vi "8.0.0_Tester_Functionality_Buyoff.vi"(8 "error in (no error)":errorcluster, 10 "?":T1, 11 "Message Queue out":T2) -> (0 "error out":errorcluster, 1 "Flow":string, 2 "Data":T1, 3 "Message Queue Out":T2)   [LabVIEW 2017]
uses:
  DIPC 692 Daemon API/typdef/calibration.ctl
  DIPC 692 Daemon API/typdef/task_detect_test_point.ctl
  DIPC 692 Daemon API/typdef/device_mode.ctl
  DIPC 692 Daemon API/typdef/destination.ctl
  Depends/AMC/subVIs/TypeDefs/amc_Message Queue.ctl
  Depends/AMC/subVIs/TypeDefs/amc_Message.ctl
  Depends/Tools/Keyed Array/Tools_KeyedArray KeyedArray.ctl
  Ctrls/Data.ctl
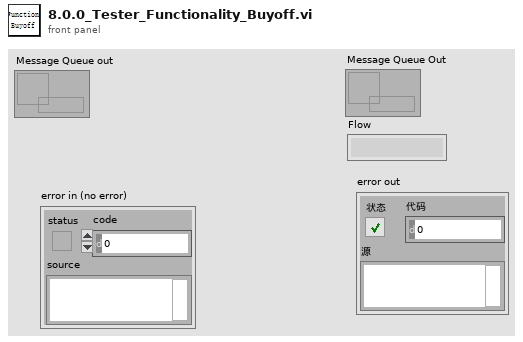
[diagram p1: front panel]
types:
  T1 = typedef "Data.ctl" = cluster{"SN":string, "Start Time":timestamp, "Step Time":timestamp, "Count":cluster{"Total":i32, "OK":i32, "NG":i32, "Yield":dbl}, "Table":string[][], "daemon reference":refnum<k5>, "CT":dbl, "Config":string[][], "Initialisation":cluster{"Set_SKU_Config_With_LMT_Error":string, "FCT_timestamp":string, "sw_version_before":string, "hardware_serial":string, "Backup_DDM_NVM":string, "Flash_SW_follow_SKU":string, "sw_version_after":string, "Set_SKU_Config_base_on_variant":string, "UUT_Ready_Status":string, "Set_DDM_to_EOL_Mode":string, "DDM_Parameter":dbl[], "DDM_Parameter_status":bool[], "Get_Tester_Parameter":dbl[], "Get_Tester_Parameter_status":bool[], "Cal_Tester_Parameter":dbl[], "Cal_Tester_Parameter_status":bool[], "sw_version_before_status":bool, "sw_version_after_status":bool, "Reflashing_Flash_SW_follow_SKU":string, "Set_SKU_Config_With_LMT_status":bool, "FCT_timestamp_status":bool, "LMT_Connect_to_UUT":string, "LMT_Read_SC_SW":string, "LMT_Write_SKU_File":string, "LMT_Connect_to_UUT_status":bool}, "BEMF_Calibration":cluster{"Read_ambient_temperature":dbl, "Set_ambient_temperature_to_DDM":string, "Save_Calibration":string, "Calibration_Vaule":dbl[], "Calibration_Start_Calibration":string, "Calibration_Vaule _B":dbl[], "Calibration_Vaule_status":bool[], "Calibration_Vaule_B_status":bool[], "Orifice_Size":string}, "ECO":cluster{"Reset_Power_tune_vaule_to_zero":string, "ECO_Motor_On_with_power_mode":string, "DDM_Parameter":dbl[], "DDM_Parameter_status":bool[], "Get_Tester_Parameter":dbl[], "Get_Tester_Parameter_status":bool[], "Cal_Tester_Parameter":dbl[], "Cal_Tester_Parameter_status":bool[], "DDM_Parameter_after_power_tune":dbl[], "Get_Tester_Parameter_after_power_tune":dbl[], "Cal_Tester_Parameter_after_power_tune":dbl[], "Cal_Tester_Parameter_after_power_tune_status":bool[], "Delta_P":dbl, "ECO_Power_Tune_Set_Delta_Power_tune_value_to_DDM":string, "ECO_Power_Tune_Motor_On_with_power_mode":string, "Reset_BEMF_FISF_calibration":string, "Orifice_Size":string}, "BOOST":cluster{"DDM_Parameter":dbl[], "DDM_Parameter_status":bool[], "Get_Tester_Parameter":dbl[], "Get_Tester_Parameter_status":bool[], "Cal_Tester_Parameter":dbl[], "Cal_Tester_Parameter_status":bool[], "DDM_Parameter_after_power_tune":dbl[], "Get_Tester_Parameter_after_power_tune":dbl[], "Cal_Tester_Parameter_after_power_tune":dbl[], "Cal_Tester_Parameter_after_power_tune_status":bool[], "airwatts_am_off":dbl, "AW_Delta_(AM_on_and_off)":dbl, "AW_Delta_(AM_on_and_off)_Status":bool, "Delta_P":dbl, "BOOST_Motor_On_with_power_mode":string, "BOOST_Air_Muscle_Check_Turn_off_air_muscle":string, "BOOST_Power_Tune_Set_Delta_Power_tune_value_to_DDM":string, "BOOST_Power_Tune_Motor_On_with_power_mode":string, "BOOST_Stop_motor":string, "BOOST_Save_Calibration":string, "BOOST_Get_AW_Calibration_value":string, "Orifice_Size":string}, "MAX":cluster{"Max_Motor_On_with_power_mode":string, "Average_Tmag_Data":cluster{"LSI Delta in degC":dbl, "FISF Delta in degc":dbl, "LSI Tmag in degC":dbl, "Fisf Tmag in degC":dbl, "IIR Tmag in degC":dbl}, "DDM_Parameter":dbl[], "DDM_Parameter_status":bool[], "Get_Tester_Parameter":dbl[], "Get_Tester_Parameter_status":bool[], "Cal_Tester_Parameter":dbl[], "BEMF_Finetune":cluster{"eol_bemf_mp_cold_coef_c":dbl, "eol_cold_bemf_fisf_offset":dbl}, "AW_Tune":cluster{"delta_P1":dbl, "delta_P_Setting":dbl}, "DDM_Parameter_after_Airwatts_Tune":dbl[], "Get_Tester_Parameter_after_Airwatts_Tune":dbl[], "Cal_Tester_Parameter_after_Airwatts_Tune":dbl[], "DDM_Parameter_after_Airwatts_Finetune":dbl[], "Get_Tester_Parameter_after_Airwatts_Finetune":dbl[], "Cal_Tester_Parameter_after_Airwatts_Finetune":dbl[], "AW_Finetune":cluster{"delta_P2":dbl, "delta_P_Setting":dbl}, "Delta_Tmag_after_tune":cluster{"LSI Delta in degC":dbl, "FISF Delta in degc":dbl, "LSI Tmag in degC":dbl, "Fisf Tmag in degC":dbl, "IIR Tmag in degC":dbl}, "Hot Bemf in mV":dbl, "DDM_Pressure":dbl, "Delta_Pressure":dbl, " Cold Bemf in mV":dbl, " delta Bemf":dbl, " delta p":dbl, "Delta_Pressure_status":bool, " delta Bemf_status":bool, "LSI Delta in degC_status":bool, "FISF Delta in degc_status":bool, "Motor_On_with_power_mode_after_Airwatts_Tune":string, "Airwatts_Finetune_Motor_On_with_power_mode":string, "Airwatts_Finetune_Stop_motor":string, "Max_check_derate_status":string, "Max_Stop_motor":string, "Max_Save_Calibration":string, "Max_check_derate_status_status":bool, "Average_All_data":dbl[][], "Average_Tmag_Data_status":bool[], "Average_Tmag_Data_after_tune_status":bool[], "Orifice_Size":string, "Cal_Tester_Parameter_status":bool[], "Cal_Tester_Parameter_status_after_Airwatts_Tune":bool[], "Cal_Tester_Parameter_status_after_Airwatts_FineTune":bool[]}, "Task_Detect_Calib":cluster{"LL":cluster{"DDM_Parameter":dbl[], "DDM_Parameter_status":bool[], "Get_Tester_Parameter":dbl[], "Get_Tester_Parameter_status":bool[], "Set_task_detect_A":dbl, "LL_Motor_On":string, "Orifice_Size":string, "Set_task_detect_A_Status":bool}, "HL":cluster{"DDM_Parameter":dbl[], "DDM_Parameter_status":bool[], "Get_Tester_Parameter":dbl[], "Get_Tester_Parameter_status":bool[], "Set_task_detect_B":dbl, "HL_Motor_On":string, "HL_Motor_Stop":string, "Set_task_detect_B_Status":bool}, "LH":cluster{"DDM_Parameter":dbl[], "DDM_Parameter_status":bool[], "Get_Tester_Parameter":dbl[], "Get_Tester_Parameter_status":bool[], "Set_task_detect_C":dbl, "LH_Motor_On":string, "Orifice_Size":string, "Set_task_detect_C_Status":bool}, "HH":cluster{"DDM_Parameter":dbl[], "DDM_Parameter_status":bool[], "Get_Tester_Parameter":dbl[], "Get_Tester_Parameter_status":bool[], "Set_task_detect_D":dbl, "HH_Motor_On":string, "HH_Set_calibration_eol_inlet_blockage":string, "HH_Motor_Stop":string, "HH_Save_calibration":string, "Read_and_check_calibration_Status":bool[], "Set_task_detect_D_Status":bool}, "Get_eol_inlet_blockage_E":dbl, "Calib_vaule":cluster{"Get_task_detect_LL":dbl, "Get_task_detect_HL":dbl, "Get_task_detect_LH":dbl, "Get_task_detect_HH":dbl, "eol_inlet_blockage":dbl, "eol_code_bemf_temp":dbl}, "Reset_all_task_detect_calibration_parameter":string, "calibrated temp":dbl, "Set ambient temperature to DDM":string, "Set ambient temperature to DDM after task detect":string, "Inlet_Blockage_Calibration":cluster{"DDM_Parameter":dbl[], "DDM_Parameter_status":bool[], "Get_Tester_Parameter":dbl[], "Get_Tester_Parameter_status":bool[], "Inlet_Blockage_Calibration_Motor_On":string, "Calibrate Inlet Blockage":string}, "Get_eol_inlet_blockage_E_Status":bool}, "good":cluster{"Write_Product_TS":cluster{"TIMESTAMP":i64, "RIG_ID":i64, "PASSMARK_ID":i64, "PASSMARK_REV":i64}, "Read_Product_TS":cluster{"TIMESTAMP":i64, "RIG_ID":i64, "PASSMARK_ID":i64, "PASSMARK_REV":i64}, "Good_Clear_NVM_Error":string, "Good_Set_DDM_to_Product_mode":string, "Good_Write_Product_Timestamp":string, "Good_Read_Product_Timestamp":string, "Good_Backup_DDM_NVM":string, "Good_Set_Secuity_Bit":string, "Good_Set_Calibration_Lock":string, "Good_Check_Secuity_Bit":string, "Good_Check_Secuity_Bit_Stauts":bool}, "UUT_Type":enum16{"692", "692B", "692D"}, "NG":cluster{"NG_Read_Error":string, "NG_Change_to_FCT_mode":string, "NG_Backup_DDM_NVM":string}, "OK/NG":bool, "Model":string, "Station ID":string}
  T2 = typedef "amc_Message Queue.ctl" = refnum<queue>
  T3 = typedef "HD Config.ctl" = cluster{" PC":cluster{"PC Address":u8[], "PC Port":i32}, "FCO":cluster{"COM":refnum<visa-resource-name>, "Baudrate":u32}, "DC Power ":cluster{"COM":refnum<visa-resource-name>, "Baudrate":u32}, "PW3336":cluster{"COM":refnum<visa-resource-name>, "Baudrate":u32}, "Lefoo":cluster{"COM":refnum<visa-resource-name>, "Baudrate":u32}, "AI Model":cluster{"COM":refnum<visa-resource-name>, "Baudrate":u32}, "DIPC":cluster{"COM":refnum<visa-resource-name>}, "Daemon":cluster{"IP Address":string, "Port":u16, "Retry":u16}, "Motor":cluster{"COM":refnum<visa-resource-name>, "Baudrate":u32}, "G1":bool, "Fail_resume_mode":bool, "Skip DDM Speed&Pressure Passmark":bool}
  T4 = typedef "destination.ctl" = string
  T5 = typedef "calibration.ctl" = string
  T6 = typedef "device_mode.ctl" = enum16{"FCT", "EOL", "PROD"}
  T7 = typedef "airwatt tune parameter.ctl" = cluster{"Index(0-5)":i64, "Target power mW":i64, "Offset power mW":i64}
  T8 = typedef "task_detect_test_point.ctl" = enum16{"LL", "HL", "LH", "HH"}
  T9 = cluster{"TIMESTAMP":i64, "RIG_ID":i64, "PASSMARK_ID":i64, "PASSMARK_REV":i64}
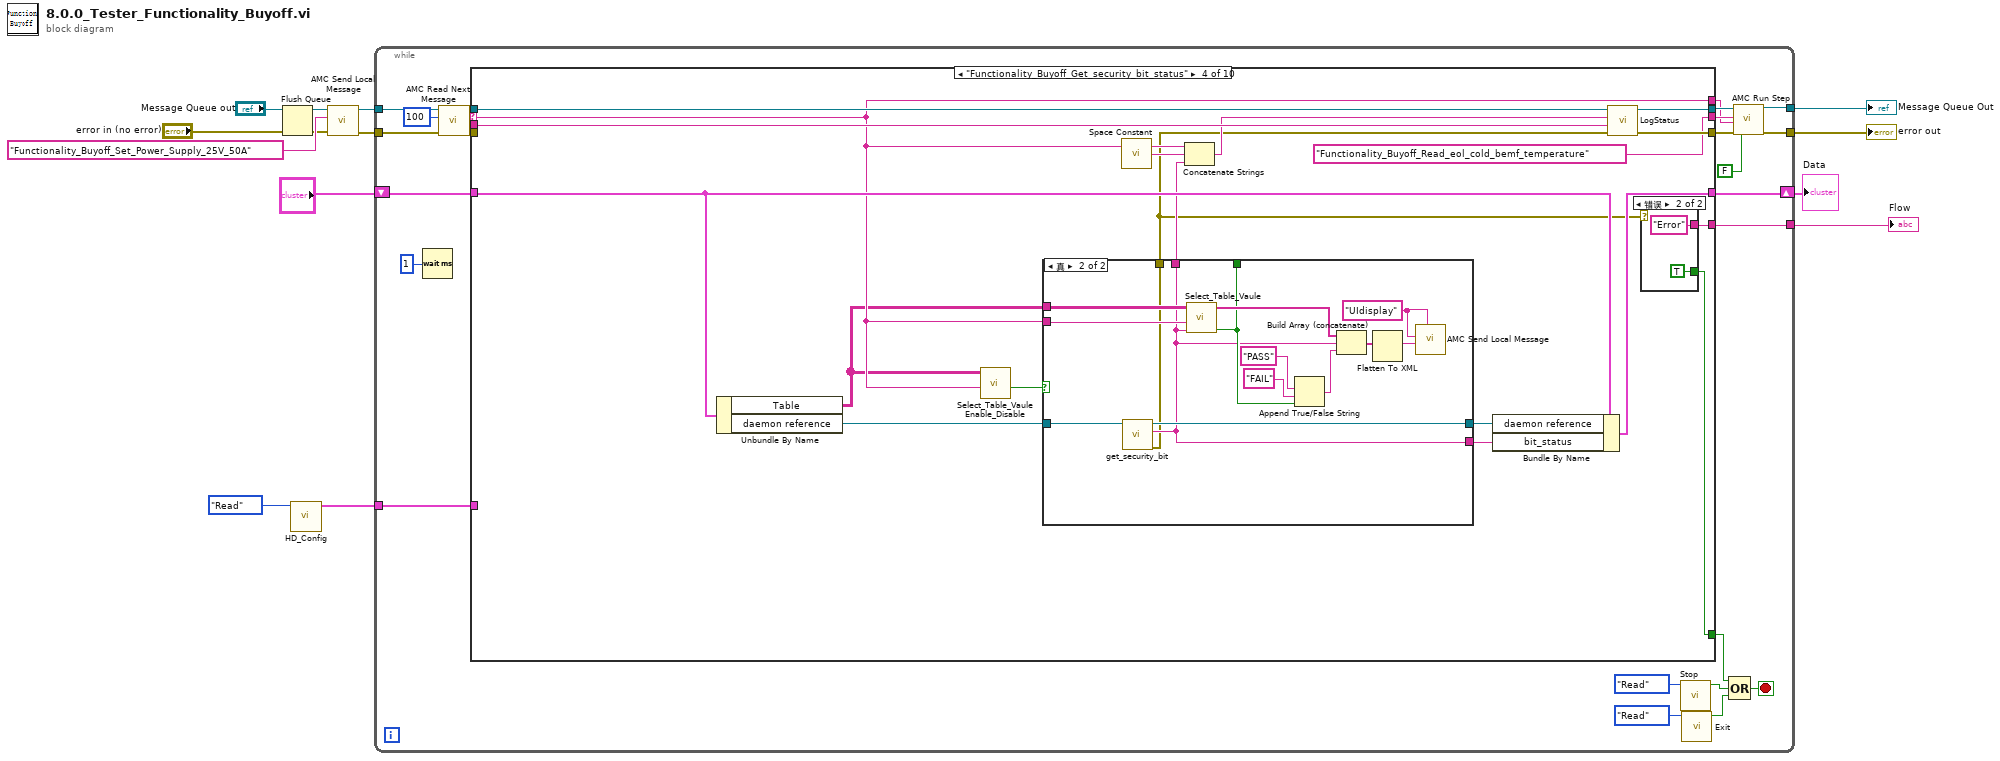
[diagram p0: block diagram]
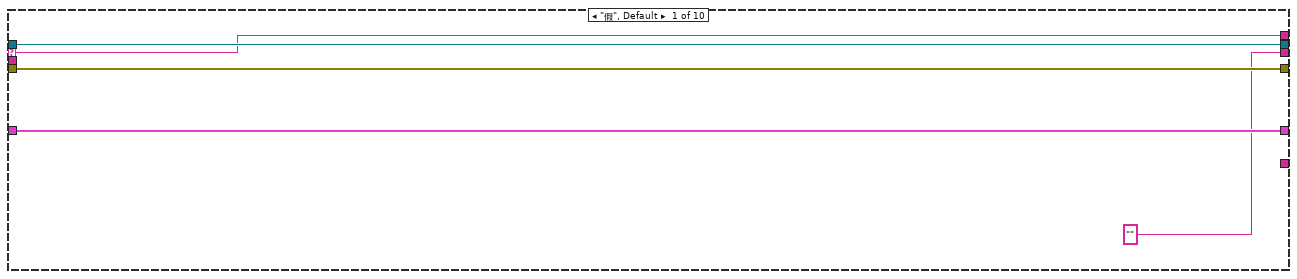
[diagram p2: hidden frame]
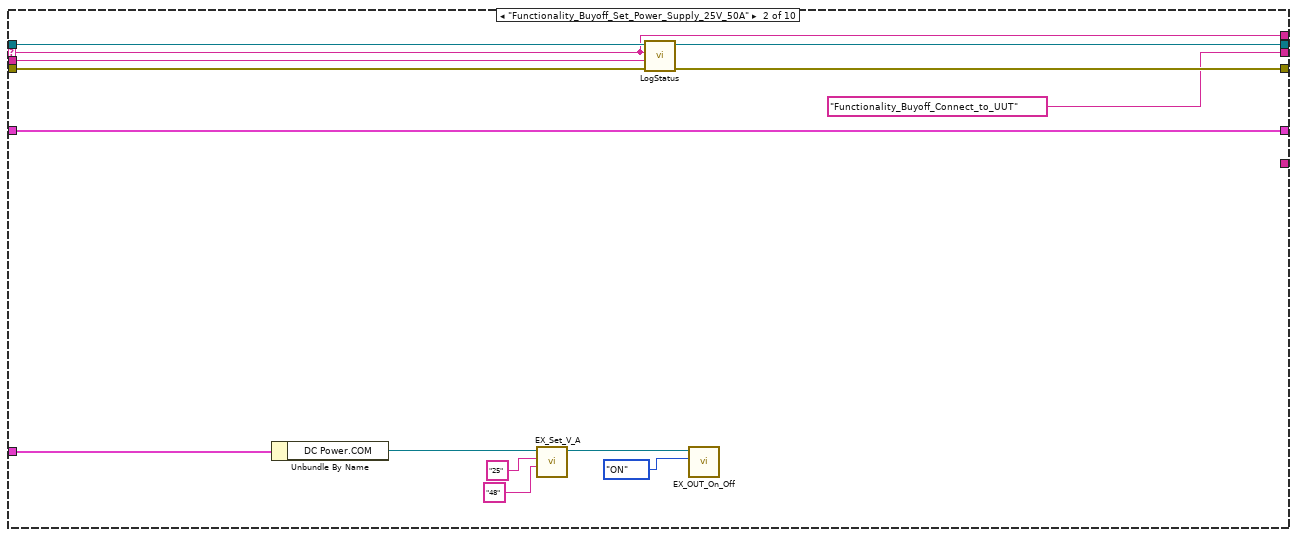
[diagram p3: hidden frame]
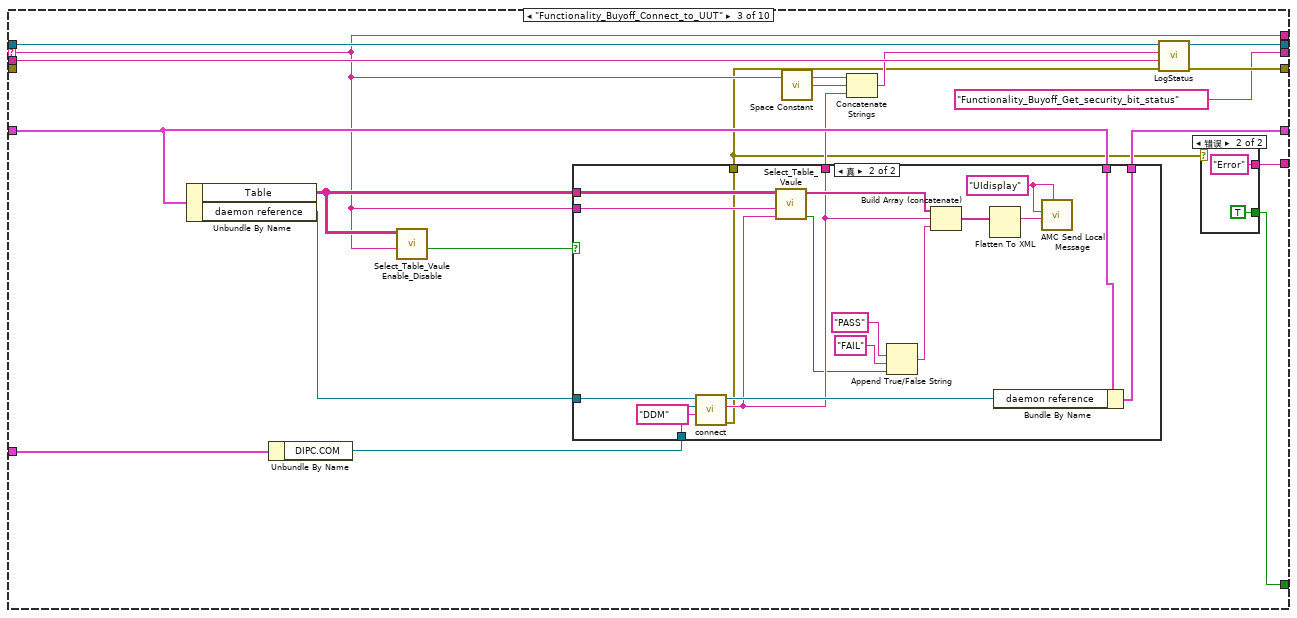
[diagram p4: hidden frame]
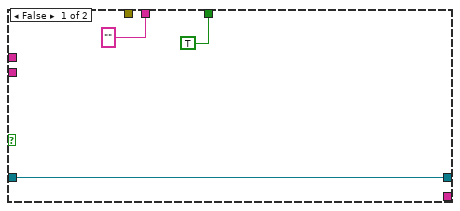
[diagram p8: hidden frame]
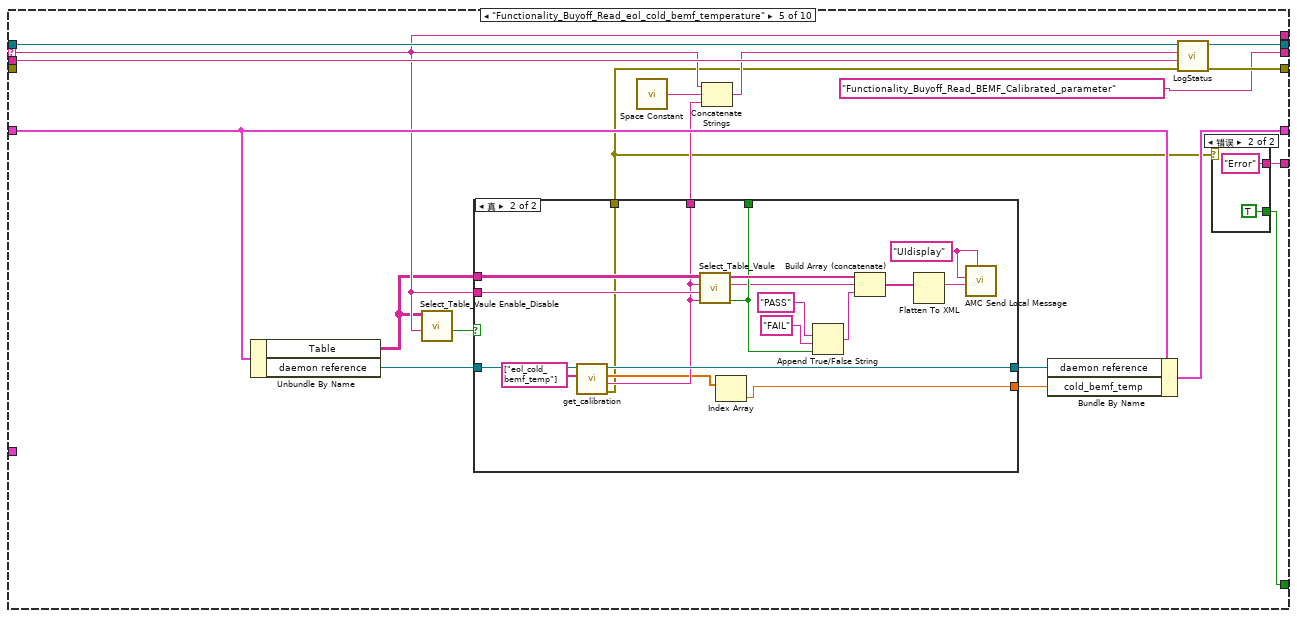
[diagram p9: hidden frame]
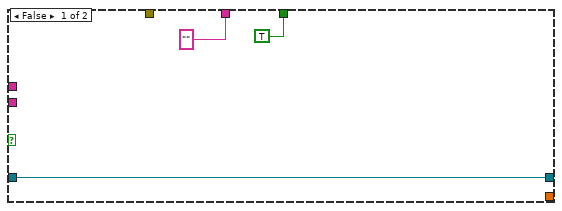
[diagram p11: hidden frame]
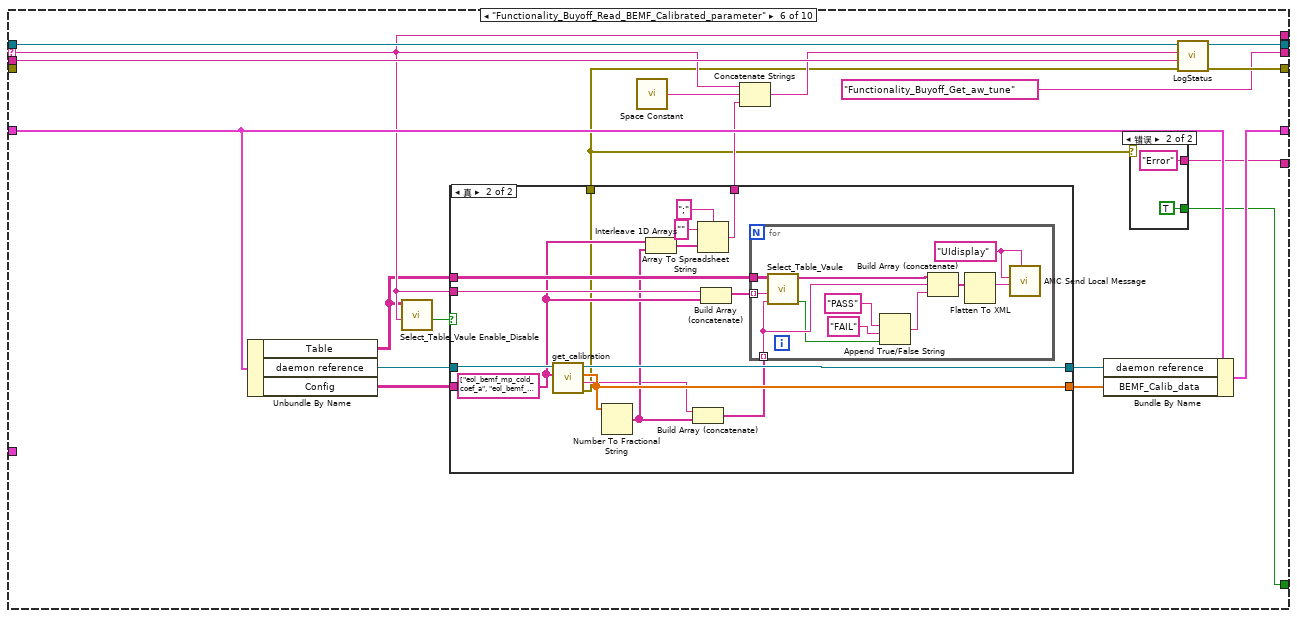
[diagram p12: hidden frame]
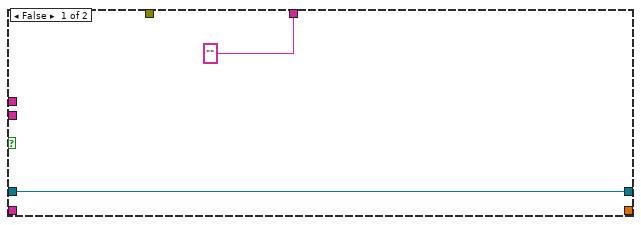
[diagram p14: hidden frame]
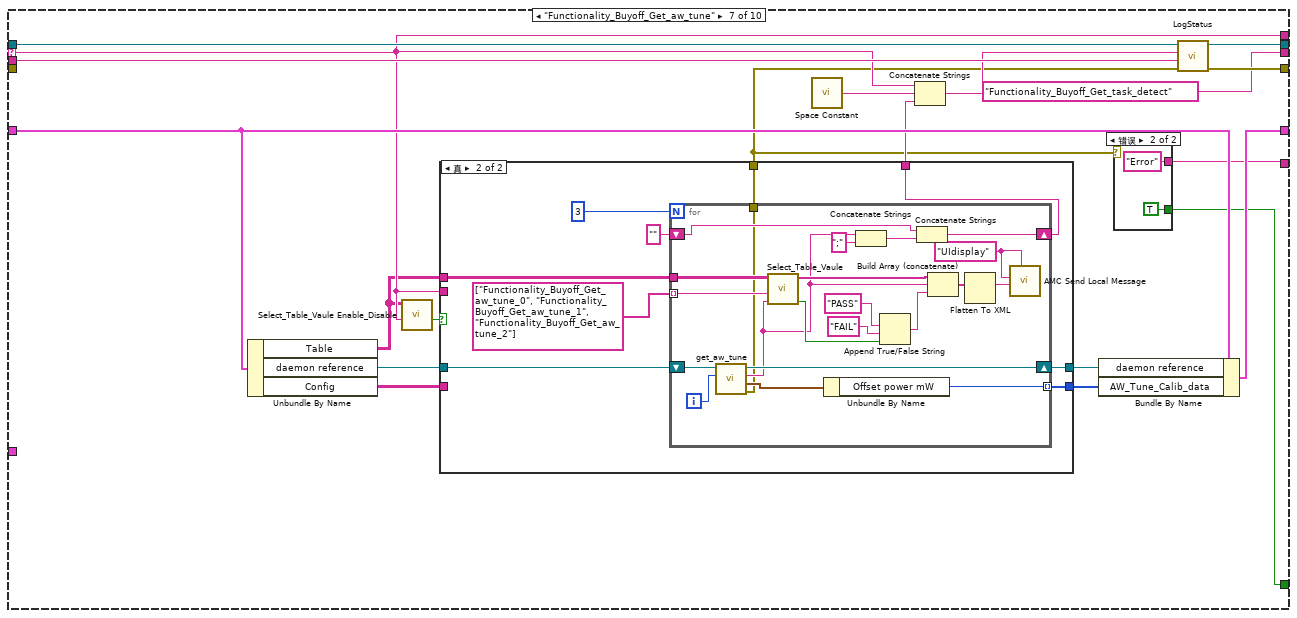
[diagram p15: hidden frame]
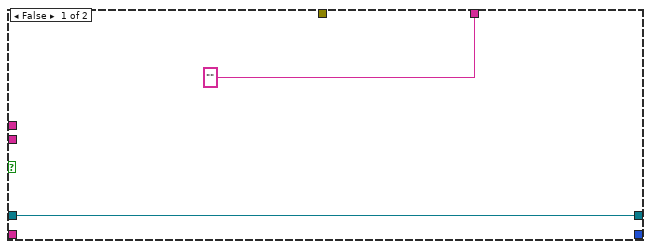
[diagram p17: hidden frame]
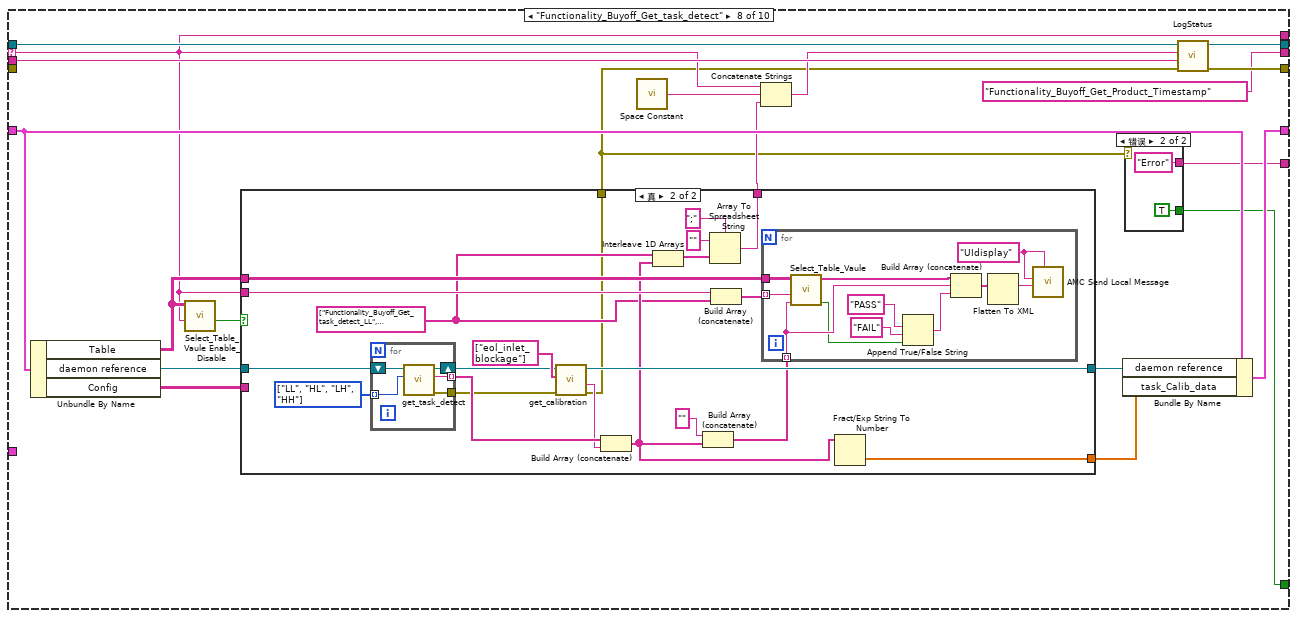
[diagram p18: hidden frame]
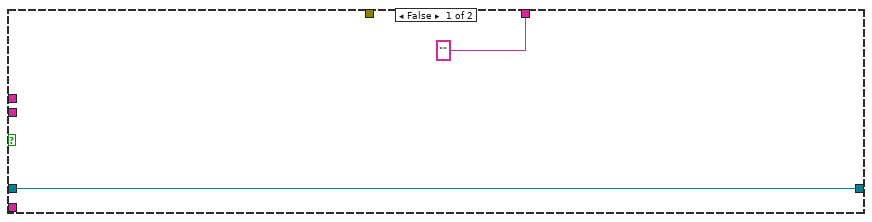
[diagram p20: hidden frame]
diagram:
  n1 = Flush Queue(queue="Message Queue out") -> (queue out=w1:T2)  [unwired: 1 in, 2 out]
  n2 = call "HD_Config.vi"("Step"=enum16{"Initial", "Write", "Read"}."Read") -> ("HD Config out"=w5:T3)  [unwired: 9 in, 1 out]
  n3 = call "AMC Send Local Message.vi"("error in (no error)"="error in (no error)", "Message Name"="Functionality_Buyoff_Set_Power_Supply_25V_50A", "Message Queue in"=w1) -> ("error out"=w10:errorcluster, "Message Queue out"=w11:T2)  [unwired: 7 in]
  n4 = while {
    tunnel: w11 -> [w38]
    tunnel: [w34] -> w3
    tunnel: w10 -> [w32]
    tunnel: [w29] -> w2
    shift-right: [w25] -> w7
    shift-left: "?" -> [w26]
    tunnel: w5 -> [w24]
    tunnel: [w20] -> w4
    stop <- w14 stop-if-true
    n5 = Wait (ms)(milliseconds to wait=u32 1 ("等待时间（毫秒）")) -> ()  [unwired: 1 out]
    n6 = call "AMC Read Next Message.vi"("error in (no error)"=w32, "timeout (1ms)"=100, "Message Queue in"=w38) -> ("error out"=w31:errorcluster, "Message Value"=w22:string, "Message Name"=w36:string, "Message Queue out"=w37:T2)  [unwired: 1 in, 4 out]
    n7 = case shown="\"Functionality_Buyoff_Get_security_bit_status\"" w36 {
      selector: w36 -> [w40 w51 w62 w102 w139 w181 w230 w281 w342 w379]
      tunnel: w37 -> [w43 w56 w74 w113 w150 w191 w240 w293 w352 w390]
      tunnel: [w43 w56 w74 w113 w150 w191 w240 w293 w352 w390] -> w35
      tunnel: w31 -> [w42 w54 _ _ _ _ _ _ _ _]
      tunnel: [w42 w53 w73 w112 w149 w190 w239 w292 w351 w389] -> w30
      tunnel: [_ _ w59 w97 w134 w174 w223 w276 w336 TRUE] -> w15
      tunnel: w26 -> [w41 w55 w67 w108 w146 w187 w236 w290 w348 w386]
      tunnel: [w41 w55 w68 w107 w145 w186 w235 w289 w347 w385] -> w25
      tunnel: w22 -> [_ w52 w72 w111 w148 w189 w238 w291 w350 w388]
      tunnel: [w40 w51 w62 w102 w139 w181 w230 w281 w342 w379] -> w21
      tunnel: w24 -> [_ w45 w70 _ _ _ _ _ _ _]
      tunnel: ["" "Functionality_Buyoff_Connect_to_UUT" "Functionality_Buyoff_Get_security_bit_status" "Functionality_Buyoff_Read_eol_cold_bemf_temperature" "Functionality_Buyoff_Read_BEMF_Calibrated_parameter" "Functionality_Buyoff_Get_aw_tune" "Functionality_Buyoff_Get_task_detect" "Functionality_Buyoff_Get_Product_Timestamp" "Functionality_Buyoff_Get_calibration_lock_status" w376] -> w23
      tunnel: [_ _ w60 w98 w135 w175 w224 w277 w338 w376] -> w20
      frame "假", Default {
      }
      frame "Functionality_Buyoff_Set_Power_Supply_25V_50A" {
        n8 = Unbundle By Name(w45) -> ("DC Power.COM"=w44:refnum<visa-resource-name>)
        n9 = call "EX_Set_V_A.vi"("current"="48", "voltage"="25", "VISA resource name"=w44) -> ("VISA资源名称输出"=w47:refnum<visa-resource-name>)  [unwired: 7 in, 1 out]
        n10 = call "LogStatus.vi"("error in (no error)"=w54, "last message"=w52, "message"=w51) -> ("error  out"=w53:errorcluster)  [unwired: 8 in]
        n11 = call "EX_OUT_On_Off.vi"("Mode"=enum16{"ON", "OFF"}."ON", "VISA resource name"=w47) -> ()  [unwired: 8 in, 2 out]
      }
      frame "Functionality_Buyoff_Connect_to_UUT" {
        n12 = Unbundle By Name(w67) -> ("Table"=w63:string[][], "daemon reference"=w57:refnum<k5>)
        n13 = Unbundle By Name(w70) -> ("DIPC.COM"=w69:refnum<visa-resource-name>)
        n14 = call "Select_Table_Vaule Enable_Disable.vi"("Action"=w62, "Table"=w63) -> ("Enable"=w61:bool)  [unwired: 8 in, 1 out]
        n15 = case shown="真" w61 {
          tunnel: w69 -> [_ w95]
          tunnel: [w77 w94] -> w68
          tunnel: w67 -> [w77 w93]
          tunnel: [_ w84] -> w64
          tunnel: w63 -> [_ w82]
          tunnel: w62 -> [_ w81]
          tunnel: [_ w80] -> w58
          tunnel: w57 -> [_ w79]
          frame False {
          }
          frame True {
            w90 = "UIdisplay" ("Process (\"\" - local)")
            n16 = call "connect.vi"("Target"=T4 "DDM", "physical connection"=w95, "daemon reference in"=w79) -> ("error out"=w80:errorcluster, "response"=w84:string, "daemon reference out"=w91:refnum<k5>)  [unwired: 4 in, 2 out]
            n17 = call "Select_Table_Vaule.vi"("Vaule"=w84, "Action"=w81, "Table"=w82) -> ("Result"=w83:bool, "vaule"=w92:string[])  [unwired: 7 in]
            n18 = Append True/False String(1:w83, 2:"FAIL" ("真字符串"), 3:"PASS" ("真字符串")) -> (0:w85:string)  [unwired: 1 in]
            n19 = Build Array (concatenate)(w92, w84, w85) -> (w89:string[])
            n20 = Flatten To XML(anything=w89) -> (xml string=w88:string)
            n21 = Bundle By Name(cluster=w93, "daemon reference"=w91) -> (w94:T1)
            n22 = call "AMC Send Local Message.vi"("Process (\"\" - local)"=w90, "Message Value"=w88, "Message Name"=w90) -> ()  [unwired: 7 in, 2 out]
          }
        }
        n23 = call <vilib>:"Space Constant.vi"() -> ("String"=w65:string)
        n24 = Concatenate Strings(w62, w65, w64) -> (w66:string)
        n25 = call "LogStatus.vi"("error in (no error)"=w58, "last message"=w72, "message"=w66) -> ("error  out"=w73:errorcluster)  [unwired: 8 in]
        n26 = case shown="错误" w58 {
          tunnel: [_ TRUE] -> w59
          tunnel: [_ "Error"] -> w60
          frame No Error {
          }
          frame Error {
          }
        }
      }
      frame "Functionality_Buyoff_Get_security_bit_status" {
        n27 = Unbundle By Name(w108) -> ("Table"=w101:string[][], "daemon reference"=w110:refnum<k5>)
        n28 = call "Select_Table_Vaule Enable_Disable.vi"("Action"=w102, "Table"=w101) -> ("Enable"=w103:bool)  [unwired: 8 in, 1 out]
        n29 = case shown="真" w103 {
          tunnel: w110 -> [w117 w132]
          tunnel: [TRUE w121] -> _
          tunnel: [w117 w125] -> w109
          tunnel: ["" ("response") w120] -> w104
          tunnel: w102 -> [_ w124]
          tunnel: w101 -> [_ w123]
          tunnel: [_ w120] -> w99
          tunnel: [_ w119] -> w96
          frame False {
          }
          frame True {
            w131 = "UIdisplay" ("Process (\"\" - local)")
            n30 = call "get_security_bit.vi"("daemon reference in"=w132) -> ("error out"=w119:errorcluster, "response"=w120:string, "daemon reference out"=w125:refnum<k5>)  [unwired: 7 in, 1 out]
            n31 = call "Select_Table_Vaule.vi"("Vaule"=w120, "Action"=w124, "Table"=w123) -> ("Result"=w121:bool, "vaule"=w122:string[])  [unwired: 7 in]
            n32 = Append True/False String(1:w121, 2:"FAIL" ("真字符串"), 3:"PASS" ("真字符串")) -> (0:w126:string)  [unwired: 1 in]
            n33 = Build Array (concatenate)(w122, w120, w126) -> (w130:string[])
            n34 = Flatten To XML(anything=w130) -> (xml string=w129:string)
            n35 = call "AMC Send Local Message.vi"("Process (\"\" - local)"=w131, "Message Value"=w129, "Message Name"=w131) -> ()  [unwired: 7 in, 2 out]
          }
        }
        n36 = call <vilib>:"Space Constant.vi"() -> ("String"=w106:string)
        n37 = Concatenate Strings(w102, w106, w104) -> (w105:string)
        n38 = Bundle By Name(cluster=w108, "daemon reference"=w109, "bit_status"=w99) -> (w107:T1)
        n39 = call "LogStatus.vi"("error in (no error)"=w96, "last message"=w111, "message"=w105) -> ("error  out"=w112:errorcluster)  [unwired: 8 in]
        n40 = case shown="错误" w96 {
          tunnel: [_ TRUE] -> w97
          tunnel: [_ "Error"] -> w98
          frame No Error {
          }
          frame Error {
          }
        }
      }
      frame "Functionality_Buyoff_Read_eol_cold_bemf_temperature" {
        n41 = Unbundle By Name(w146) -> ("Table"=w138:string[][], "daemon reference"=w147:refnum<k5>)
        n42 = call "Select_Table_Vaule Enable_Disable.vi"("Action"=w139, "Table"=w138) -> ("Enable"=w140:bool)  [unwired: 8 in, 1 out]
        n43 = case shown="真" w140 {
          tunnel: w147 -> [w154 w166]
          tunnel: [TRUE w161] -> _
          tunnel: [w154 w165] -> w144
          tunnel: ["" ("software string") w159] -> w141
          tunnel: w139 -> [_ w164]
          tunnel: w138 -> [_ w163]
          tunnel: [_ w157] -> w136
          tunnel: [_ w156] -> w133
          frame False {
          }
          frame True {
            w172 = "UIdisplay" ("Process (\"\" - local)")
            n44 = call "get_calibration.vi"("Calibration"=T5[] ["eol_cold_bemf_temp"], "daemon reference in"=w166) -> ("error out"=w156:errorcluster, "response"=w159:string, "values"=w158:dbl[], "daemon reference out"=w165:refnum<k5>)  [unwired: 5 in, 1 out]
            n45 = call "Select_Table_Vaule.vi"("Vaule"=w159, "Action"=w164, "Table"=w163) -> ("Result"=w161:bool, "vaule"=w162:string[])  [unwired: 7 in]
            n46 = Index Array(array=w158) -> (element=w157:dbl)  [unwired: 1 in]
            n47 = Append True/False String(1:w161, 2:"FAIL" ("真字符串"), 3:"PASS" ("真字符串")) -> (0:w167:string)  [unwired: 1 in]
            n48 = Build Array (concatenate)(w162, w159, w167) -> (w171:string[])
            n49 = Flatten To XML(anything=w171) -> (xml string=w170:string)
            n50 = call "AMC Send Local Message.vi"("Process (\"\" - local)"=w172, "Message Value"=w170, "Message Name"=w172) -> ()  [unwired: 7 in, 2 out]
          }
        }
        n51 = call <vilib>:"Space Constant.vi"() -> ("String"=w143:string)
        n52 = Concatenate Strings(w139, w143, w141) -> (w142:string)
        n53 = Bundle By Name(cluster=w146, "daemon reference"=w144, "cold_bemf_temp"=w136) -> (w145:T1)
        n54 = call "LogStatus.vi"("error in (no error)"=w133, "last message"=w148, "message"=w142) -> ("error  out"=w149:errorcluster)  [unwired: 8 in]
        n55 = case shown="错误" w133 {
          tunnel: [_ TRUE] -> w134
          tunnel: [_ "Error"] -> w135
          frame No Error {
          }
          frame Error {
          }
        }
      }
      frame "Functionality_Buyoff_Read_BEMF_Calibrated_parameter" {
        n56 = Unbundle By Name(w187) -> ("Table"=w180:string[][], "daemon reference"=w188:refnum<k5>, "Config"=w178:string[][])
        n57 = call "Select_Table_Vaule Enable_Disable.vi"("Action"=w181, "Table"=w180) -> ("Enable"=w179:bool)  [unwired: 8 in, 1 out]
        n58 = case shown="真" w179 {
          tunnel: w188 -> [w195 w209]
          tunnel: [w195 w208] -> w185
          tunnel: ["" ("software string") w199] -> w182
          tunnel: w181 -> [_ w206]
          tunnel: w180 -> [_ w210]
          tunnel: w178 -> [_ _]
          tunnel: [_ w207] -> w176
          tunnel: [_ w196] -> w173
          frame False {
          }
          frame True {
            w204 = T5[] ["eol_bemf_mp_cold_coef_a", "eol_bemf_mp_cold_coef_b", "eol_bemf_mp_cold_coef_c", "eol_bemf_lsi_cold_ref_coeffs", "eol_bemf_lsi_speed", "eol_bemf_lsi_integral_0", "eol_bemf_lsi_integral_1", "eol_bemf_lsi_integral_2", "eol_cold_bemf", "eol_cold_bemf_fisf", "eol_cold_bemf_fisf_offset"] ("Calibration")
            n59 = call "get_calibration.vi"("Calibration"=w204, "daemon reference in"=w209) -> ("error out"=w196:errorcluster, "response"=w201:string, "values"=w207:dbl[], "daemon reference out"=w208:refnum<k5>)  [unwired: 5 in, 1 out]
            n60 = Number To Fractional String(number=w207) -> (F-format string=w203:string[])  [unwired: 3 in]
            n61 = Interleave 1D Arrays(w204, w203) -> (w200:T5[])
            n62 = Build Array (concatenate)(w201, w203) -> (w202:string[])
            n63 = Array To Spreadsheet String(delimiter (Tab)=";" ("分隔符(Tab)"), array=w200, 3:"" ("格式字符串")) -> (spreadsheet string=w199:string)
            n64 = Build Array (concatenate)(w206, w204) -> (w205:T5[])
            n65 = for {
              tunnel: w210 -> [w215]
              tunnel: w202 -> [w213] mode=indexing
              tunnel: w205 -> [w212] mode=indexing
              w221 = "UIdisplay" ("Process (\"\" - local)")
              n66 = call "Select_Table_Vaule.vi"("Vaule"=w213, "Action"=w212, "Table"=w215) -> ("Result"=w211:bool, "vaule"=w214:string[])  [unwired: 7 in]
              n67 = Append True/False String(1:w211, 2:"FAIL" ("真字符串"), 3:"PASS" ("真字符串")) -> (0:w216:string)  [unwired: 1 in]
              n68 = Build Array (concatenate)(w214, w213, w216) -> (w220:string[])
              n69 = Flatten To XML(anything=w220) -> (xml string=w219:string)
              n70 = call "AMC Send Local Message.vi"("Process (\"\" - local)"=w221, "Message Value"=w219, "Message Name"=w221) -> ()  [unwired: 7 in, 2 out]
            }
          }
        }
        n71 = call <vilib>:"Space Constant.vi"() -> ("String"=w184:string)
        n72 = Concatenate Strings(w181, w184, w182) -> (w183:string)
        n73 = Bundle By Name(cluster=w187, "daemon reference"=w185, "BEMF_Calib_data"=w176) -> (w186:T1)
        n74 = case shown="错误" w173 {
          tunnel: [_ TRUE] -> w174
          tunnel: [_ "Error"] -> w175
          frame No Error {
          }
          frame Error {
          }
        }
        n75 = call "LogStatus.vi"("error in (no error)"=w173, "last message"=w189, "message"=w183) -> ("error  out"=w190:errorcluster)  [unwired: 8 in]
      }
      frame "Functionality_Buyoff_Get_aw_tune" {
        n76 = Unbundle By Name(w236) -> ("Table"=w229:string[][], "daemon reference"=w237:refnum<k5>, "Config"=w227:string[][])
        n77 = call "Select_Table_Vaule Enable_Disable.vi"("Action"=w230, "Table"=w229) -> ("Enable"=w228:bool)  [unwired: 8 in, 1 out]
        n78 = case shown="真" w228 {
          tunnel: w237 -> [w244 w252]
          tunnel: [w244 w251] -> w234
          tunnel: ["" ("software string") w246] -> w231
          tunnel: w230 -> [_ _]
          tunnel: w229 -> [_ w253]
          tunnel: w227 -> [_ _]
          tunnel: [_ w248] -> w225
          tunnel: [_ w245] -> w222
          frame False {
          }
          frame True {
            n79 = for {
              N: 3 -> [_]
              tunnel: w253 -> [w274]
              shift-right: [w272] -> w251
              shift-left: w252 -> [w273]
              tunnel: string[] ["Functionality_Buyoff_Get_aw_tune_0", "Functionality_Buyoff_Get_aw_tune_1", "Functionality_Buyoff_Get_aw_tune_2"] -> [w262] mode=indexing
              tunnel: [w260] -> w248 mode=indexing
              shift-right: [w257] -> w246
              shift-left: "" -> [w256]
              tunnel: [w254] -> w245
              i -> [w263]
              w271 = "UIdisplay" ("Process (\"\" - local)")
              n80 = call "get_aw_tune.vi"("Index"=w263, "daemon reference in"=w273) -> ("error out"=w254:errorcluster, "AW Tune Parameter"=w261:T7, "response"=w259:string, "daemon reference out"=w272:refnum<k5>)  [unwired: 5 in, 1 out]
              n81 = call "Select_Table_Vaule.vi"("Vaule"=w259, "Action"=w262, "Table"=w274) -> ("Result"=w264:bool, "vaule"=w265:string[])  [unwired: 7 in]
              n82 = Unbundle By Name(w261) -> ("Offset power mW"=w260:i64)
              n83 = Concatenate Strings(w259, ";" ("字符串")) -> (w255:string)
              n84 = Append True/False String(1:w264, 2:"FAIL" ("真字符串"), 3:"PASS" ("真字符串")) -> (0:w266:string)  [unwired: 1 in]
              n85 = Concatenate Strings(w256, w255) -> (w257:string)
              n86 = Build Array (concatenate)(w265, w259, w266) -> (w270:string[])
              n87 = Flatten To XML(anything=w270) -> (xml string=w269:string)
              n88 = call "AMC Send Local Message.vi"("Process (\"\" - local)"=w271, "Message Value"=w269, "Message Name"=w271) -> ()  [unwired: 7 in, 2 out]
            }
          }
        }
        n89 = call <vilib>:"Space Constant.vi"() -> ("String"=w233:string)
        n90 = Concatenate Strings(w230, w233, w231) -> (w232:string)
        n91 = Bundle By Name(cluster=w236, "daemon reference"=w234, "AW_Tune_Calib_data"=w225) -> (w235:T1)
        n92 = case shown="错误" w222 {
          tunnel: [_ TRUE] -> w223
          tunnel: [_ "Error"] -> w224
          frame No Error {
          }
          frame Error {
          }
        }
        n93 = call "LogStatus.vi"("error in (no error)"=w222, "last message"=w238, "message"=w232) -> ("error  out"=w239:errorcluster)  [unwired: 8 in]
      }
      frame "Functionality_Buyoff_Get_task_detect" {
        n94 = Unbundle By Name(w290) -> ("Table"=w282:string[][], "daemon reference"=w284:refnum<k5>, "Config"=w283:string[][])
        n95 = call "Select_Table_Vaule Enable_Disable.vi"("Action"=w281, "Table"=w282) -> ("Enable"=w285:bool)  [unwired: 8 in, 1 out]
        n96 = case shown="真" w285 {
          tunnel: w284 -> [w297 w317]
          tunnel: [w297 w306] -> w280
          tunnel: ["" ("software string") w311] -> w279
          tunnel: w281 -> [_ w315]
          tunnel: w282 -> [_ w318]
          tunnel: [_ w302] -> w278
          tunnel: w283 -> [_ _]
          tunnel: [_ w298] -> w275
          frame False {
          }
          frame True {
            w300 = string[] ["Functionality_Buyoff_Get_task_detect_LL", "Functionality_Buyoff_Get_task_detect_HL", "Functionality_Buyoff_Get_task_detect_LH", "Functionality_Buyoff_Get_task_detect_HH", "Functionality_Buyoff_Get_calibration_eol_inlet_blockage"]
            w310 = T8[] [enum."LL", enum."HL", enum."LH", enum."HH"] items=["LL", "HL", "LH", "HH"]
            n97 = for {
              tunnel: [w321] -> w305 mode=indexing
              shift-right: [w322] -> w307
              shift-left: w317 -> [w323]
              tunnel: w310 -> [w320] mode=indexing
              tunnel: [w319] -> w299
              n98 = call "get_task_detect.vi"("Test Point"=w320, "daemon reference in"=w323) -> ("error out"=w319:errorcluster, "response"=w321:string, "daemon reference out"=w322:refnum<k5>)  [unwired: 6 in, 1 out]
            }
            n99 = call "get_calibration.vi"("error in (no error)"=w299, "Calibration"=T5[] ["eol_inlet_blockage"], "daemon reference in"=w307) -> ("error out"=w298:errorcluster, "response"=w304:string, "daemon reference out"=w306:refnum<k5>)  [unwired: 4 in, 2 out]
            n100 = Build Array (concatenate)(w305, w304) -> (w301:string[])
            n101 = Interleave 1D Arrays(w300, w301) -> (w314:string[])
            n102 = Build Array (concatenate)("", w301) -> (w303:string[])
            n103 = Array To Spreadsheet String(delimiter (Tab)=";" ("格式字符串"), array=w314, 3:"" ("格式字符串")) -> (spreadsheet string=w311:string)
            n104 = Build Array (concatenate)(w315, w300) -> (w316:string[])
            n105 = for {
              tunnel: w318 -> [w328]
              tunnel: w303 -> [w326] mode=indexing
              tunnel: w316 -> [w325] mode=indexing
              w334 = "UIdisplay" ("Process (\"\" - local)")
              n106 = call "Select_Table_Vaule.vi"("Vaule"=w326, "Action"=w325, "Table"=w328) -> ("Result"=w324:bool, "vaule"=w327:string[])  [unwired: 7 in]
              n107 = Append True/False String(1:w324, 2:"FAIL" ("真字符串"), 3:"PASS" ("真字符串")) -> (0:w329:string)  [unwired: 1 in]
              n108 = Build Array (concatenate)(w327, w326, w329) -> (w333:string[])
              n109 = Flatten To XML(anything=w333) -> (xml string=w332:string)
              n110 = call "AMC Send Local Message.vi"("Process (\"\" - local)"=w334, "Message Value"=w332, "Message Name"=w334) -> ()  [unwired: 7 in, 2 out]
            }
            n111 = Fract/Exp String To Number(string=w301) -> (number=w302:dbl[])  [unwired: 3 in, 1 out]
          }
        }
        n112 = call <vilib>:"Space Constant.vi"() -> ("String"=w288:string)
        n113 = Concatenate Strings(w281, w288, w279) -> (w287:string)
        n114 = Bundle By Name(cluster=w290, "daemon reference"=w280, "task_Calib_data"=w278) -> (w289:T1)
        n115 = case shown="错误" w275 {
          tunnel: [_ TRUE] -> w276
          tunnel: [_ "Error"] -> w277
          frame No Error {
          }
          frame Error {
          }
        }
        n116 = call "LogStatus.vi"("error in (no error)"=w275, "last message"=w291, "message"=w287) -> ("error  out"=w292:errorcluster)  [unwired: 8 in]
      }
      frame "Functionality_Buyoff_Get_Product_Timestamp" {
        n117 = Unbundle By Name(w348) -> ("Table"=w341:string[][], "daemon reference"=w349:refnum<k5>)
        n118 = call "Select_Table_Vaule Enable_Disable.vi"("Action"=w342, "Table"=w341) -> ("Enable"=w343:bool)  [unwired: 8 in, 1 out]
        n119 = case shown="真" w343 {
          tunnel: w349 -> [w356 w367]
          tunnel: [TRUE w362] -> _
          tunnel: [w356 w366] -> w346
          tunnel: ["" ("software string") w361] -> w335
          tunnel: w342 -> [_ w365]
          tunnel: w341 -> [_ w364]
          tunnel: [_ w359] -> w339
          tunnel: [_ w358] -> w337
          frame False {
          }
          frame True {
            w373 = "UIdisplay" ("Process (\"\" - local)")
            n120 = call "get_cal_info.vi"("Mode"=device_mode."PROD", "daemon reference in"=w367) -> ("error out"=w358:errorcluster, "Parameter"=w359:T9, "response"=w361:string, "daemon reference out"=w366:refnum<k5>)  [unwired: 5 in, 1 out]
            n121 = call "Select_Table_Vaule.vi"("Vaule"=w361, "Action"=w365, "Table"=w364) -> ("Result"=w362:bool, "vaule"=w363:string[])  [unwired: 7 in]
            n122 = Append True/False String(1:w362, 2:"FAIL" ("真字符串"), 3:"PASS" ("真字符串")) -> (0:w368:string)  [unwired: 1 in]
            n123 = Build Array (concatenate)(w363, w361, w368) -> (w372:string[])
            n124 = Flatten To XML(anything=w372) -> (xml string=w371:string)
            n125 = call "AMC Send Local Message.vi"("Process (\"\" - local)"=w373, "Message Value"=w371, "Message Name"=w373) -> ()  [unwired: 7 in, 2 out]
          }
        }
        n126 = call <vilib>:"Space Constant.vi"() -> ("String"=w345:string)
        n127 = Concatenate Strings(w342, w345, w335) -> (w344:string)
        n128 = Bundle By Name(cluster=w348, "Functionality_Buyoff_Get_Product_Timestamp"=w335, "daemon reference"=w346, "good.Read_Product_TS"=w339) -> (w347:T1)
        n129 = case shown="错误" w337 {
          tunnel: [_ TRUE] -> w336
          tunnel: [_ "Error"] -> w338
          frame No Error {
          }
          frame Error {
          }
        }
        n130 = call "LogStatus.vi"("error in (no error)"=w337, "last message"=w350, "message"=w344) -> ("error  out"=w351:errorcluster)  [unwired: 8 in]
      }
      frame "Functionality_Buyoff_Get_calibration_lock_status" {
        n131 = Unbundle By Name(w386) -> ("Table"=w378:string[][], "daemon reference"=w387:refnum<k5>)
        n132 = call "Select_Table_Vaule Enable_Disable.vi"("Action"=w379, "Table"=w378) -> ("Enable"=w380:bool)  [unwired: 8 in, 1 out]
        n133 = case shown="真" w380 {
          tunnel: w387 -> [w394 w403]
          tunnel: [TRUE w398] -> _
          tunnel: [w394 w402] -> w384
          tunnel: ["" ("software string") w397] -> w381
          tunnel: w379 -> [_ w401]
          tunnel: w378 -> [_ w400]
          tunnel: [_ w397] -> w377
          tunnel: [_ w396] -> w374
          frame False {
          }
          frame True {
            w409 = "UIdisplay" ("Process (\"\" - local)")
            n134 = call "get_calibration_lock.vi"("daemon reference in"=w403) -> ("error out"=w396:errorcluster, "response"=w397:string, "daemon reference out"=w402:refnum<k5>)  [unwired: 7 in, 1 out]
            n135 = call "Select_Table_Vaule.vi"("Vaule"=w397, "Action"=w401, "Table"=w400) -> ("Result"=w398:bool, "vaule"=w399:string[])  [unwired: 7 in]
            n136 = Append True/False String(1:w398, 2:"FAIL" ("真字符串"), 3:"PASS" ("真字符串")) -> (0:w404:string)  [unwired: 1 in]
            n137 = Build Array (concatenate)(w399, w397, w404) -> (w408:string[])
            n138 = Flatten To XML(anything=w408) -> (xml string=w407:string)
            n139 = call "AMC Send Local Message.vi"("Process (\"\" - local)"=w409, "Message Value"=w407, "Message Name"=w409) -> ()  [unwired: 7 in, 2 out]
          }
        }
        n140 = call <vilib>:"Space Constant.vi"() -> ("String"=w383:string)
        n141 = Concatenate Strings(w379, w383, w381) -> (w382:string)
        n142 = case shown="错误" w374 {
          tunnel: ["Disconnect_UUT" "Error"] -> w376
          frame No Error {
          }
          frame Error {
          }
        }
        n143 = Bundle By Name(cluster=w386, "daemon reference"=w384, "lock_status"=w377) -> (w385:T1)
        n144 = call "LogStatus.vi"("error in (no error)"=w374, "last message"=w388, "message"=w382) -> ("error  out"=w389:errorcluster)  [unwired: 8 in]
      }
    }
    n145 = call "Stop.vi"("Step"=enum16{"Initial", "Write", "Read"}."Read") -> ("Stop Out"=w17:bool)  [unwired: 9 in, 1 out]
    n146 = call "Exit.vi"("Step"=enum16{"Initial", "Write", "Read"}."Read" ("step")) -> ("Exit Out"=w16:bool)  [unwired: 9 in, 1 out]
    n147 = Compound Arithmetic op=OR(w15, w17, w16) -> (w14:bool)
    n148 = call "AMC Run Step.vi"("Message Queue In"=w35, "Message Name"=w23, "Message Value"=w21, "error in (no error)"=w30, "Mli/Sig"=FALSE) -> ("Message Queue Out"=w34:T2, "error out"=w29:errorcluster)  [unwired: 13 in]
  }
  "Message Queue Out" <- w3
  "error out" <- w2
  "Data" <- w7
  "Flow" <- w4
